vi "arm_delta.vi"(8 "Compliance [V]":dbl=0.5 format="%#_6f", 9 "DELAY [sec]":dbl=0.002 format="%#_6e", 10 "I-HIGH [A]":dbl=0.0001 format="%#_6e") -> ()   [LabVIEW 2013]
panel:
  out "error out":errorcluster
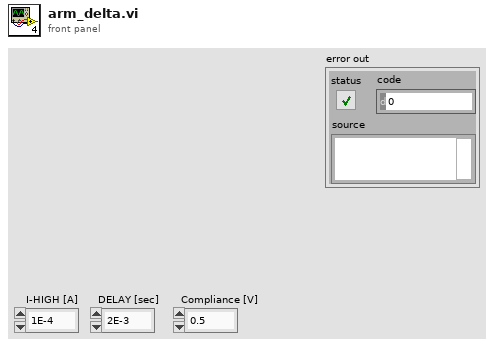
[diagram p1: front panel]
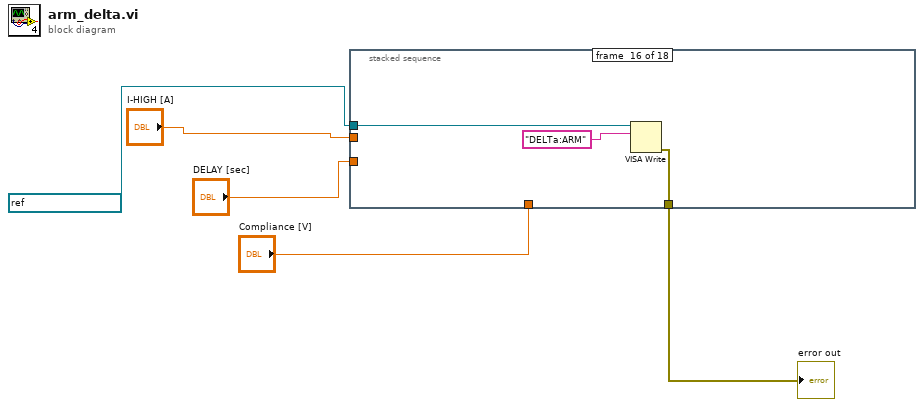
[diagram p0: block diagram]
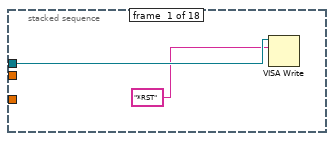
[diagram p2: hidden frame]
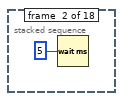
[diagram p3: hidden frame]
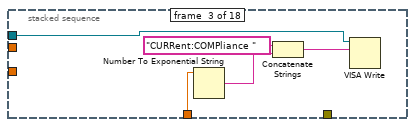
[diagram p4: hidden frame]
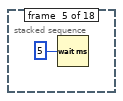
[diagram p6: hidden frame]
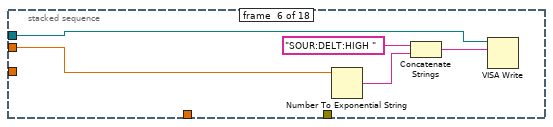
[diagram p7: hidden frame]
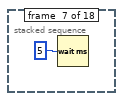
[diagram p8: hidden frame]
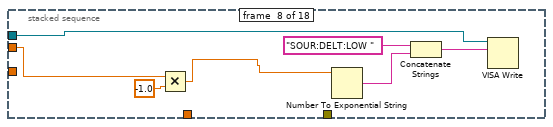
[diagram p9: hidden frame]
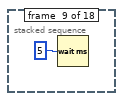
[diagram p10: hidden frame]
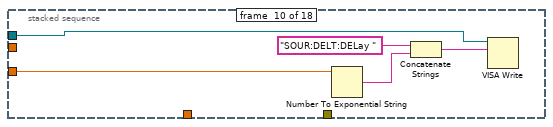
[diagram p11: hidden frame]
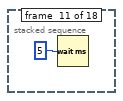
[diagram p12: hidden frame]
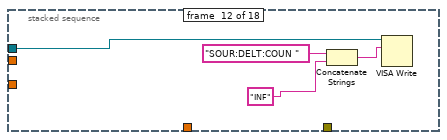
[diagram p13: hidden frame]
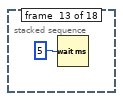
[diagram p14: hidden frame]
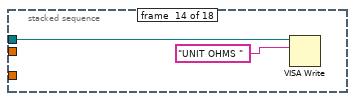
[diagram p15: hidden frame]
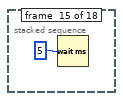
[diagram p16: hidden frame]
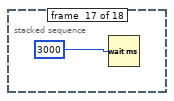
[diagram p17: hidden frame]
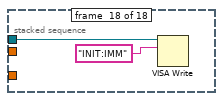
[diagram p18: hidden frame]
diagram:
  n1 = stacked-sequence {
    tunnel: "I-HIGH [A]" -> [_ _ _ _ _ w17 _ w21 _ _ _ _ _ _ _ _ _ _]
    tunnel: refnum<visa-resource-name> "GPIB0::20::INSTR" ("Keithley") -> [w7 _ w10 _ _ w15 _ w24 _ w30 _ w35 _ w40 _ w44 _ w47]
    tunnel: "DELAY [sec]" -> [_ _ _ _ _ _ _ _ _ w29 _ _ _ _ _ _ _ _]
    tunnel: "Compliance [V]" -> [_ _ w9 _ _ _ _ _ _ _ _ _ _ _ _ _ _ _]
    tunnel: [_ _ _ _ _ _ _ _ _ _ _ _ _ _ _ w43 _ _] -> w1
    frame #0 {
      n2 = VISA Write(VISA resource name=w7, write buffer="*RST") -> ()  [unwired: 1 in, 3 out]
    }
    frame #1 {
      n3 = Wait (ms)(milliseconds to wait=5) -> ()  [unwired: 1 out]
    }
    frame #2 {
      n4 = Number To Exponential String(number=w9) -> (E-format string=w12:string)  [unwired: 3 in]
      n5 = Concatenate Strings("CURRent:COMPliance ", w12) -> (w11:string)
      n6 = VISA Write(VISA resource name=w10, write buffer=w11) -> ()  [unwired: 1 in, 3 out]
    }
    frame #3 {
    }
    frame #4 {
      n7 = Wait (ms)(milliseconds to wait=5) -> ()  [unwired: 1 out]
    }
    frame #5 {
      n8 = Number To Exponential String(number=w17) -> (E-format string=w18:string)  [unwired: 3 in]
      n9 = Concatenate Strings("SOUR:DELT:HIGH ", w18) -> (w16:string)
      n10 = VISA Write(VISA resource name=w15, write buffer=w16) -> ()  [unwired: 1 in, 3 out]
    }
    frame #6 {
      n11 = Wait (ms)(milliseconds to wait=5) -> ()  [unwired: 1 out]
    }
    frame #7 {
      n12 = Multiply(x=w21, y=-1.0) -> (x*y=w22:dbl)
      n13 = Number To Exponential String(number=w22) -> (E-format string=w26:string)  [unwired: 3 in]
      n14 = Concatenate Strings("SOUR:DELT:LOW ", w26) -> (w25:string)
      n15 = VISA Write(VISA resource name=w24, write buffer=w25) -> ()  [unwired: 1 in, 3 out]
    }
    frame #8 {
      n16 = Wait (ms)(milliseconds to wait=5) -> ()  [unwired: 1 out]
    }
    frame #9 {
      n17 = Number To Exponential String(number=w29) -> (E-format string=w32:string)  [unwired: 3 in]
      n18 = Concatenate Strings("SOUR:DELT:DELay ", w32) -> (w31:string)
      n19 = VISA Write(VISA resource name=w30, write buffer=w31) -> ()  [unwired: 1 in, 3 out]
    }
    frame #10 {
      n20 = Wait (ms)(milliseconds to wait=5) -> ()  [unwired: 1 out]
    }
    frame #11 {
      n21 = Concatenate Strings("SOUR:DELT:COUN ", "INF") -> (w37:string)
      n22 = VISA Write(VISA resource name=w35, write buffer=w37) -> ()  [unwired: 1 in, 3 out]
    }
    frame #12 {
      n23 = Wait (ms)(milliseconds to wait=5) -> ()  [unwired: 1 out]
    }
    frame #13 {
      n24 = VISA Write(VISA resource name=w40, write buffer="UNIT OHMS ") -> ()  [unwired: 1 in, 3 out]
    }
    frame #14 {
      n25 = Wait (ms)(milliseconds to wait=5) -> ()  [unwired: 1 out]
    }
    frame #15 {
      n26 = VISA Write(VISA resource name=w44, write buffer="DELTa:ARM") -> (error out=w43:errorcluster)  [unwired: 1 in, 2 out]
    }
    frame #16 {
      n27 = Wait (ms)(milliseconds to wait=3000) -> ()  [unwired: 1 out]
    }
    frame #17 {
      n28 = VISA Write(VISA resource name=w47, write buffer="INIT:IMM") -> ()  [unwired: 1 in, 3 out]
    }
  }
  "error out" <- w1
